vi "Generate TCP Error.vi"(0 "VI Name":string, 7 "TCP response code":i32) -> (15 "error out":errorcluster)   [LabVIEW 2020, in "epl-network.lvlib"]
uses:
  epl-network.lvlib
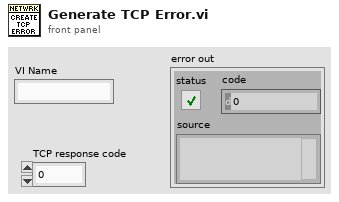
[diagram p1: front panel]
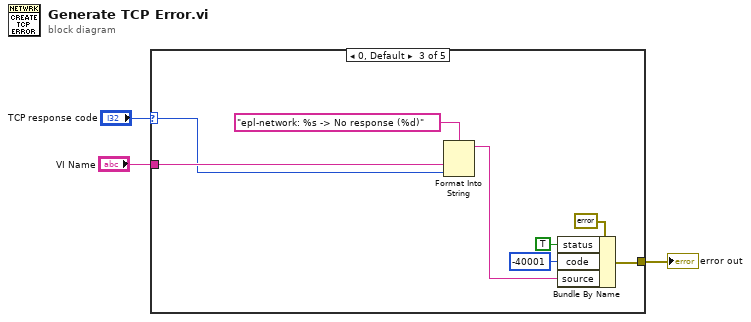
[diagram p0: block diagram]
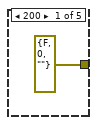
[diagram p2: hidden frame]
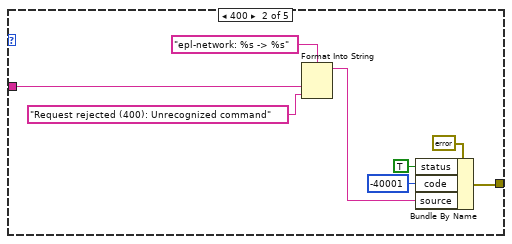
[diagram p3: hidden frame]
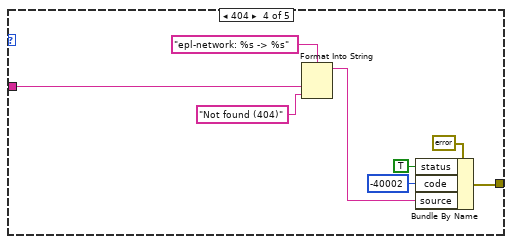
[diagram p4: hidden frame]
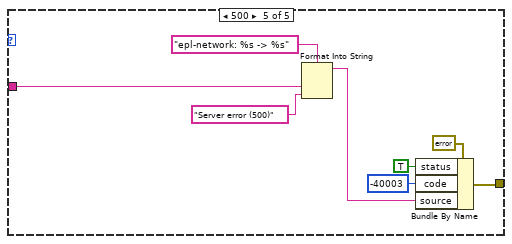
[diagram p5: hidden frame]
diagram:
  n1 = case shown="0, Default" "TCP response code" {
    selector: "TCP response code" -> [_ _ w13 _ _]
    tunnel: [errorcluster {"status"=FALSE, "code"=0, "source"=""} ("error constant") w9 w17 w25 w33] -> w3
    tunnel: "VI Name" -> [_ w7 w15 w23 w31]
    frame 200 {
    }
    frame 400 {
      n2 = Format Into String(format string="epl-network: %s -> %s", w7, "Request rejected (400): Unrecognized command" ("input 2")) -> (resulting string=w6:string)  [unwired: 2 in, 1 out]
      n3 = Bundle By Name(cluster=errorcluster {"status"=FALSE, "code"=0, "source"=""} ("error constant"), "status"=TRUE, "code"=-40001, "source"=w6) -> (w9:errorcluster)
    }
    frame 0, Default {
      n4 = Format Into String(format string="epl-network: %s -> No response (%d)", w15, w13) -> (resulting string=w14:string)  [unwired: 2 in, 1 out]
      n5 = Bundle By Name(cluster=errorcluster {"status"=FALSE, "code"=0, "source"=""} ("error constant"), "status"=TRUE, "code"=-40001, "source"=w14) -> (w17:errorcluster)
    }
    frame 404 {
      n6 = Format Into String(format string="epl-network: %s -> %s", w23, "Not found (404)" ("input 2")) -> (resulting string=w22:string)  [unwired: 2 in, 1 out]
      n7 = Bundle By Name(cluster=errorcluster {"status"=FALSE, "code"=0, "source"=""} ("error constant"), "status"=TRUE, "code"=-40002, "source"=w22) -> (w25:errorcluster)
    }
    frame 500 {
      n8 = Format Into String(format string="epl-network: %s -> %s", w31, "Server error (500)" ("input 2")) -> (resulting string=w30:string)  [unwired: 2 in, 1 out]
      n9 = Bundle By Name(cluster=errorcluster {"status"=FALSE, "code"=0, "source"=""} ("error constant"), "status"=TRUE, "code"=-40003, "source"=w30) -> (w33:errorcluster)
    }
  }
  "error out" <- w3
